vi "Initialize.vi"(8 "error in (no error)":errorcluster, 9 "Reset (True)":bool=TRUE, 10 "ID Query (True)":bool=TRUE, 11 "VISA resource name":refnum<visa-resource-name>) -> (0 "error out":errorcluster, 3 "VISA resource name out":refnum<visa-resource-name>)   [LabVIEW 2011, in "Agilent E5052X.lvlib"]
doc: "Establishes communication with the instrument and optionally performs an instrument identification query and/or an instrument reset. It also places the instrument in a default state needed for other instrument driver operations. Therefore, call this VI before calling other instrument driver VIs for this instrument. Generally, you need to call the Initialize VI only once at the beginning of an application."
uses:
  Agilent E5052X.lvlib
  <vilib>/regexp/Match Regular Expression.xnode
panel:
  # "(c) 2007-2015 National Instruments.  ALL RIGHTS RESERVED."
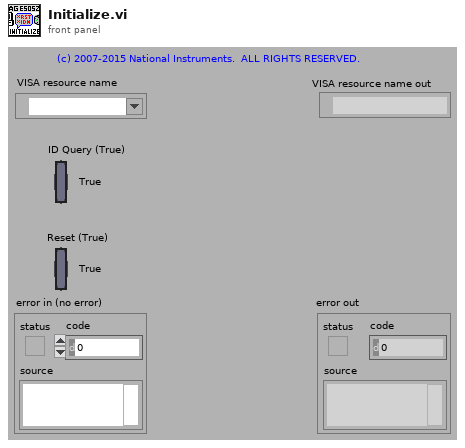
[diagram p1: front panel]
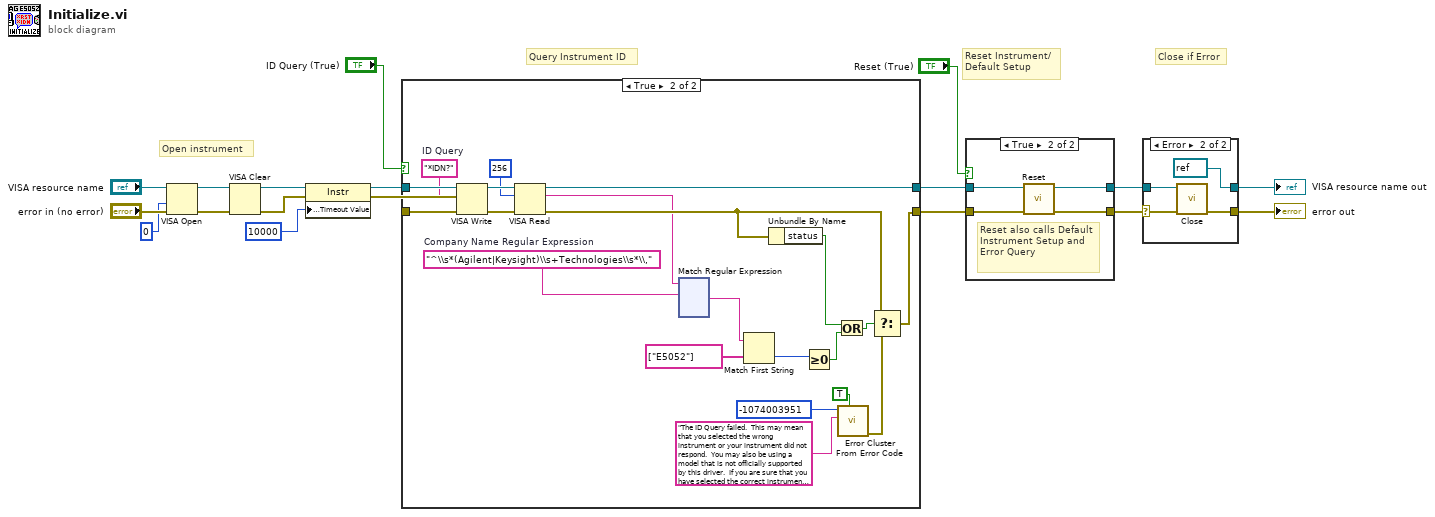
[diagram p0: block diagram]
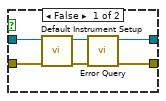
[diagram p3: hidden frame]
diagram:
  # "Close if Error"
  # "Query Instrument ID"
  # "Reset Instrument/\nDefault Setup"
  # "Open instrument"
  n1 = VISA Open(access mode=u32 0, error in (no error)="error in (no error)", VISA resource name="VISA resource name") -> (VISA resource name=w8:refnum<visa-resource-name>, error out=w7:errorcluster)  [unwired: 2 in]
  n2 = VISA Clear(VISA resource name=w8, error in (no error)=w7) -> (VISA resource name out=w6:refnum<visa-resource-name>, error out=w5:errorcluster)
  n3 = property class="Instr"(reference=w6, error in=w5, "General Settings:Timeout Value"=u32 10000) -> (reference out=w11:refnum<visa-resource-name>, error out=w10:errorcluster)
  n4 = case shown="True" "ID Query (True)" {
    tunnel: [w19 w41] -> w17
    tunnel: [w20 w38] -> w18
    tunnel: w11 -> [w20 w39]
    tunnel: w10 -> [w19 w40]
    frame False {
    }
    frame True {
      w23 = "^\\s*(Agilent|Keysight)\\s+Technologies\\s*\\,"  # Company Name Regular Expression
      w34 = "*IDN?"  # ID Query
      n5 = VISA Write(VISA resource name=w39, write buffer=w34, error in (no error)=w40) -> (VISA resource name out=w37:refnum<visa-resource-name>, error out=w36:errorcluster)  [unwired: 1 out]
      n6 = VISA Read(VISA resource name=w37, byte count=u32 256, error in (no error)=w36) -> (VISA resource name out=w38:refnum<visa-resource-name>, read buffer=w22:string, error out=w28:errorcluster)  [unwired: 1 out]
      n7 = xnode "Match Regular Expression"("input string"=w22, "regular expression"=w23) -> ("after match"=w21:string)  [unwired: 4 in, 4 out]
      n8 = Match First String(2:string[] ["E5052"] ("string array"), 3:w21) -> (0:w29:i32)  [unwired: 1 out]
      n9 = Unbundle By Name(w28) -> ("status"=w27:bool)
      n10 = Greater Or Equal To 0?(x=w29) -> (x >= 0?=w26:bool)
      n11 = Or(x=w27, y=w26) -> (x .or. y?=w25:bool)
      n12 = call <vilib>:"Error Cluster From Error Code.vi"("show call chain? (False)"=TRUE, "error message (\"\")"="The ID Query failed.  This may mean that you selected the wrong instrument or your instrument did not respond.  You may also be using a model that is not officially supported by this driver.  If you are sure that you have selected the correct instrument and it is responding, try disabling the ID Query." ("Source (VI Name)"), "error code (0)"=-1074003951 ("Code")) -> ("error out"=w33:errorcluster)  [unwired: 6 in]
      n13 = Select(t=w28, s=w25, f=w33) -> (s? t:f=w41:errorcluster)
    }
  }
  n14 = case shown="True" "Reset (True)" {
    tunnel: w17 -> [w160 w162]
    tunnel: [w157 w165] -> w1
    tunnel: w18 -> [w161 w163]
    tunnel: [w158 w164] -> w2
    frame False {
      n15 = call "Default Instrument Setup.vi"("error in (no error)"=w160, "VISA resource name"=w161) -> ("error out"=w156:errorcluster, "VISA resource name out"=w159:refnum<visa-resource-name>)  [unwired: 8 in]
      n16 = call "Error Query.vi"("error in (no error)"=w156, "VISA resource name"=w159) -> ("error out"=w157:errorcluster, "VISA resource name out"=w158:refnum<visa-resource-name>)  [unwired: 6 in, 2 out]
    }
    frame True {
      # "Reset also calls Default Instrument Setup and Error Query"
      n17 = call "Reset.vi"("error in (no error)"=w162, "VISA resource name"=w163) -> ("error out"=w165:errorcluster, "VISA resource name out"=w164:refnum<visa-resource-name>)  [unwired: 8 in]
    }
  }
  n18 = case shown="Error" w1 {
    selector: w1 -> [w166 w169]
    tunnel: w2 -> [w167 w170]
    tunnel: [w167 refnum<visa-resource-name> refnum ("VISA resource name out")] -> w4
    tunnel: [w166 w171] -> w3
    frame No Error {
    }
    frame Error {
      n19 = call "Close.vi"("error in (no error)"=w169, "VISA resource name"=w170) -> ("error out"=w171:errorcluster)  [unwired: 9 in]
    }
  }
  "VISA resource name out" <- w4
  "error out" <- w3
